vi "testUTF-8SpecialCharacters.vi"(8 "error in (no error)":errorcluster, 11 "TestCase in":refnum<class "EasyXMLTest.lvclass">) -> (0 "error out":errorcluster, 3 "TestCase out":refnum<class "EasyXMLTest.lvclass">)   [LabVIEW 2013, in "EasyXMLTest.lvclass"]
doc: "Verify that error in is not overwritten"
uses:
  EasyXMLTest.lvclass
panel:
  out "Produced Data":variant
  out "Input Data":variant
  out "XML String":string
  out "Generated XML String":string
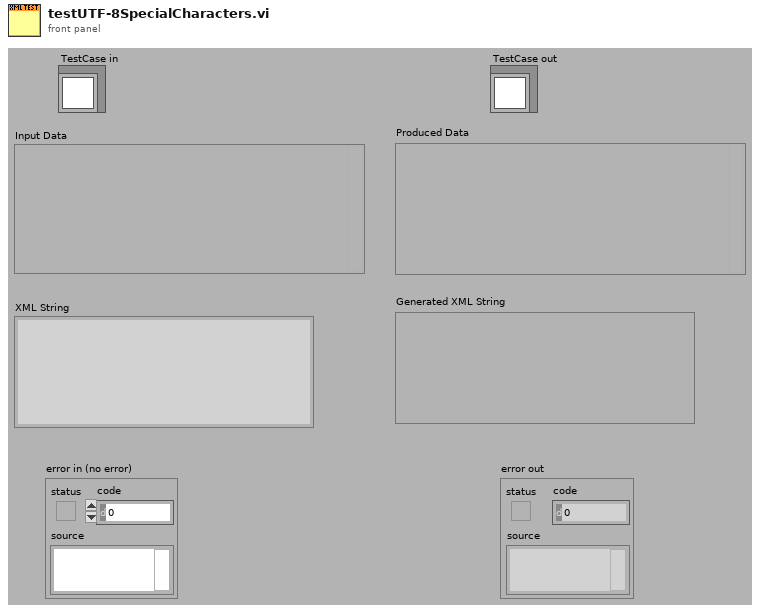
[diagram p1: front panel]
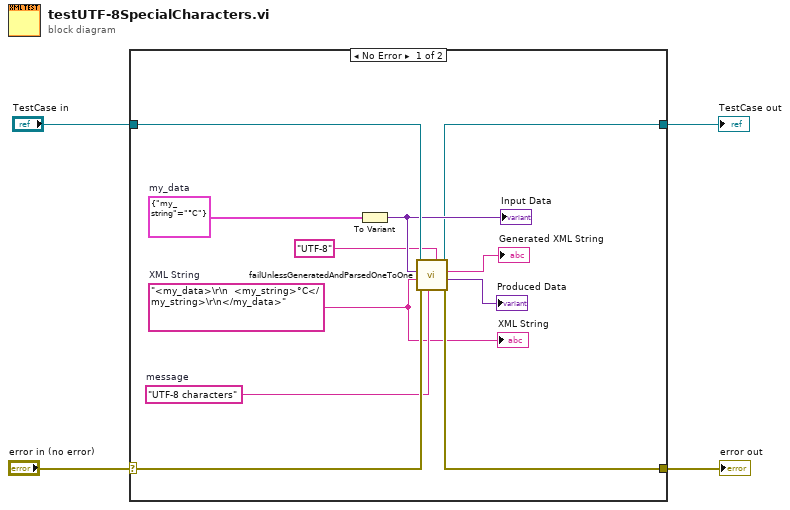
[diagram p0: block diagram]
diagram:
  n1 = case shown="No Error" "error in (no error)" {
    selector: "error in (no error)" -> [w14 w17]
    tunnel: [w9 w17] -> w2
    tunnel: [w8 w16] -> w1
    tunnel: "TestCase in" -> [w15 w16]
    frame No Error {
      w6 = cluster{"my_string":string} {"my_string"="°C"}  # my_data
      w7 = "<my_data>\r\n  <my_string>°C</my_string>\r\n</my_data>"  # XML String
      w13 = "UTF-8 characters"  # message
      n2 = To Variant(anything=w6) -> (Variant=w11:variant)
      "Input Data" <- w11
      n3 = call "failUnlessGeneratedAndParsedOneToOne.vi"("Encoding (none)"="UTF-8", "message (\"\")"=w13, "error in"=w14, "XML String"=w7, "Data"=w11, "EasyXMLTest in"=w15) -> ("error out"=w9:errorcluster, "Produced Data"=→"Produced Data":variant, "Generated XML String"=→"Generated XML String":string, "EasyXMLTest out"=w8:refnum<class "EasyXMLTest.lvclass">)  [unwired: 2 in]
      "XML String" <- w7
    }
    frame Error {
    }
  }
  "error out" <- w2
  "TestCase out" <- w1
